vi "Fit Plot to Circle.vi"(6 "Full Circle Plot":bool=TRUE, 8 "Error In":errorcluster, 11 "Circle Fit Plot Information":T2={"XY Graph Ref"=refnum, "Mouse Coordinates"={"X"=0.0, "Y"=0.0}, "Plot Index"=-1}) -> (0 "Error Out":errorcluster, 1 "Result String":string, 3 "Plot Name":string)   [LabVIEW 2019]
uses:
  <vilib>/Utility/miscctls.llb/LVPointDoubleTypeDef.ctl
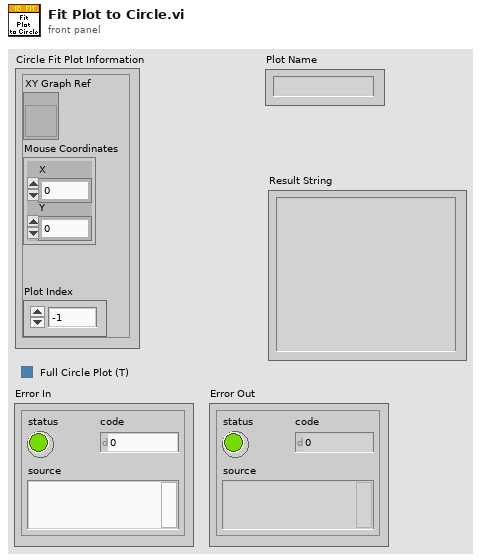
[diagram p1: front panel]
types:
  T1 = typedef "LVPointDoubleTypeDef.ctl" = cluster{"X":dbl, "Y":dbl}
  T2 = cluster{"XY Graph Ref":refnum<vi>, "Mouse Coordinates":T1, "Plot Index":i32}
  T3 = typedef "XY Graph Add-Ons.lvlib/XY Graph Refnum.ctl" = refnum<vi>
  T4 = typedef "Fitted Circle Parameters.ctl" = cluster{"x0":dbl, "y0":dbl, "r":dbl, "chi 2":dbl, "mse":dbl}
  T5 = cluster{"Fitted X Array":dbl[], "Fitted Y Array":dbl[]}
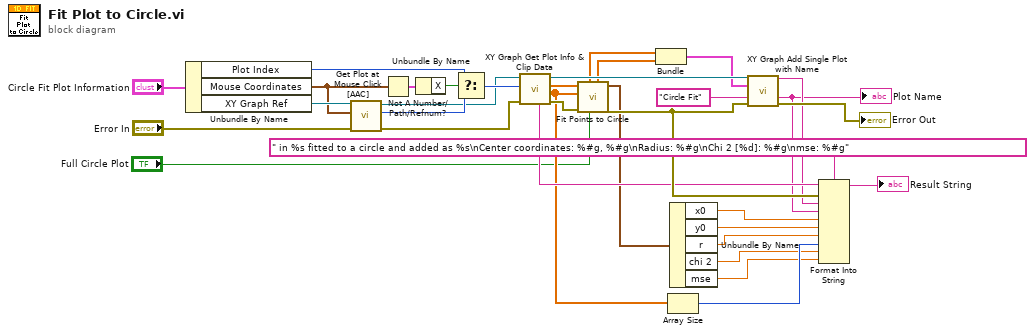
[diagram p0: block diagram]
diagram:
  n1 = Unbundle By Name("Circle Fit Plot Information") -> ("Plot Index"=w31:i32, "Mouse Coordinates"=w29:T1, "XY Graph Ref"=w30:refnum<vi>)
  n2 = call "Get Plot at Mouse Click [AAC].vi"("error in (no error)"="Error In", "Mouse Click Coordinates"=w29, "XYGraph Ref"=w30) -> ("error out"=w24:errorcluster, "Plot at Coordinates"=w27:i32, "XYGraph Ref"=w25:T3)  [unwired: 2 in, 4 out]
  n3 = Not A Number/Path/Refnum?(number/path/refnum=w29) -> (NaN/Path/Refnum?=w32:cluster{"X":bool, "Y":bool})
  n4 = Unbundle By Name(w32) -> ("X"=w33:bool)
  n5 = Select(t=w31, s=w33, f=w27) -> (s? t:f=w26:i32)
  n6 = call "XY Graph Get Plot Info & Clip Data.vi"("error in (no error)"=w24, "Plot index"=w26, "XYGraph Ref in"=w25) -> ("error out"=w22:errorcluster, "Y Array"=w9:dbl[], "X Array"=w23:dbl[], "XYGraph Ref out"=w21:refnum<vi>, "Plot Name"=w13:string)  [unwired: 3 in, 1 out]
  n7 = call "Fit Points to Circle.vi"("Full Circle Plot"="Full Circle Plot", "Error In"=w22, "Y Array"=w9, "X Array"=w23) -> ("Error Out"=w15:errorcluster, "Fitted Circle Parameters"=w7:T4, "Fitted Y Array"=w19:dbl[], "Fitted X Array"=w20:dbl[])  [unwired: 4 in]
  n8 = Bundle("Fitted X Array"=w20, "Fitted Y Array"=w19) -> (w18:T5)  [unwired: 1 in]
  n9 = Array Size(array=w9) -> (size(s)=w8:i32)
  n10 = Unbundle By Name(w7) -> ("x0"=w6:dbl, "y0"=w5:dbl, "r"=w4:dbl, "chi 2"=w3:dbl, "mse"=w2:dbl)
  n11 = call "XY Graph Add Single Plot with Name.vi"("XYGraph Ref in"=w21, "Plot"=w18, "Plot Name (\"Plot\")"="Circle Fit" ("Plot Name (\"Plot\")"), "error in (no error)"=w15) -> ("XY Graph Caption (or Label)"=w11:string, "Plot Name"=w10:string, "error out"=→"Error Out":errorcluster)  [unwired: 8 in, 1 out]
  "Plot Name" <- w10
  n12 = Format Into String(format string=" in %s fitted to a circle and added as %s\nCenter coordinates: %#g, %#g\nRadius: %#g\nChi 2 [%d]: %#g\nmse: %#g", initial string=w13, error in=w15, w11, w10, w6, w5, w4, w8, w3, w2) -> (resulting string=→"Result String":string)  [unwired: 1 out]
